vi "DAQmx.44xx.Get DAQ Type from Product Type.vi"(11 "ProductType":string) -> (3 "DAQ Type":T1)   [LabVIEW 2019, in "DAQmx.lvclass"]
uses:
  DAQmx.lvclass
  typedefs/DAQ.Config.Device Type--enum.ctl
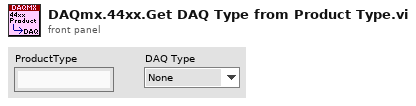
[diagram p1: front panel]
types:
  T1 = typedef "DAQmx.lvclass/DAQ.Config.Device Type--enum.ctl" = enum16{"None", "USB-4431", "PXI-446x"}
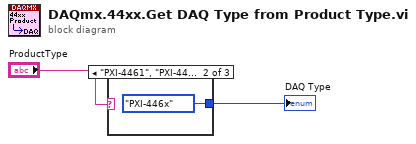
[diagram p0: block diagram]
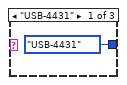
[diagram p2: hidden frame]
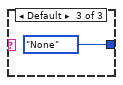
[diagram p3: hidden frame]
diagram:
  n1 = case shown="\"PXI-4461\", \"PXI-4462\"" "ProductType" {
    tunnel: [DAQ.Config.Device_Type--enum."USB-4431" ("DAQ Type") DAQ.Config.Device_Type--enum."PXI-446x" ("DAQ Type") DAQ.Config.Device_Type--enum."None" ("DAQ Type")] -> w2
    frame "USB-4431" {
    }
    frame "PXI-4461", "PXI-4462" {
    }
    frame Default {
    }
  }
  "DAQ Type" <- w2
